vi "Get Path.vi"(8 "error in (no error)":errorcluster, 11 "PathMsg in":refnum<class "PathMessage.lvclass">) -> (0 "error out":errorcluster, 2 "Message Data":path, 3 "PathMsg out":refnum<class "PathMessage.lvclass">)   [LabVIEW 2009, in "LapDog.Messaging.v2.NativeTypes.lvlib" / "PathMessage.lvclass"]
doc: "Returns the data contained in the message.\n\nThis method executes regardless of the error in state."
uses:
  PathMessage.lvclass
  PathMessage.lvclass/PathMessage.ctl
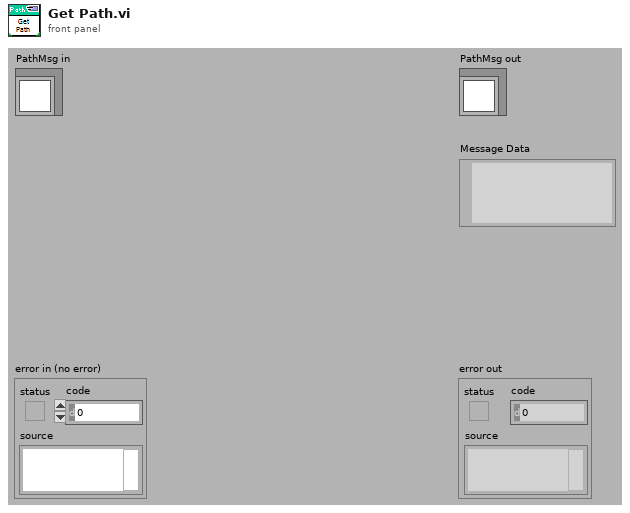
[diagram p1: front panel]
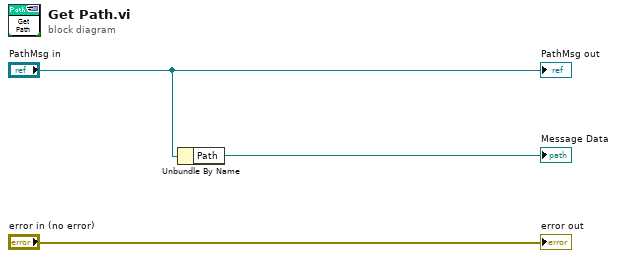
[diagram p0: block diagram]
diagram:
  n1 = Unbundle By Name("PathMsg in") -> ("Path"=→"Message Data":path)
  "error out" <- "error in (no error)"
  "PathMsg out" <- "PathMsg in"
